vi "Jacobian_h.vi"(1 "State":T1) -> (0 "J_h(H_n)":dbl[](array[numeric]))   [LabVIEW 2019]
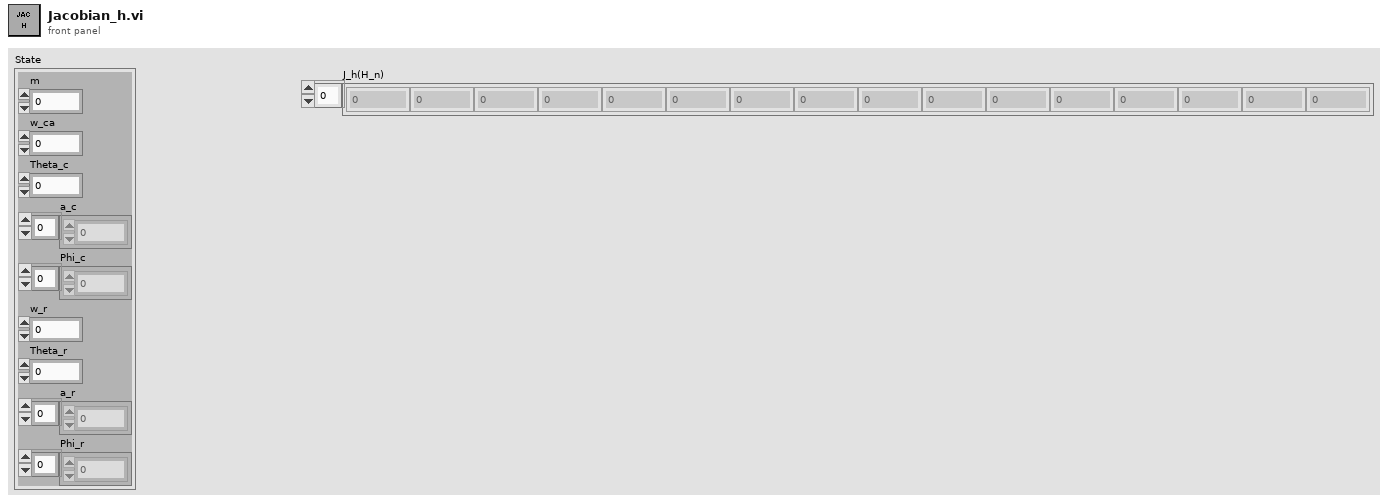
[diagram p1: front panel]
types:
  T1 = cluster{"m":dbl, "w_ca":dbl, "Theta_c":dbl, "a_c":dbl[], "Phi_c":dbl[], "w_r":dbl, "Theta_r":dbl, "a_r":dbl[], "Phi_r":dbl[]}
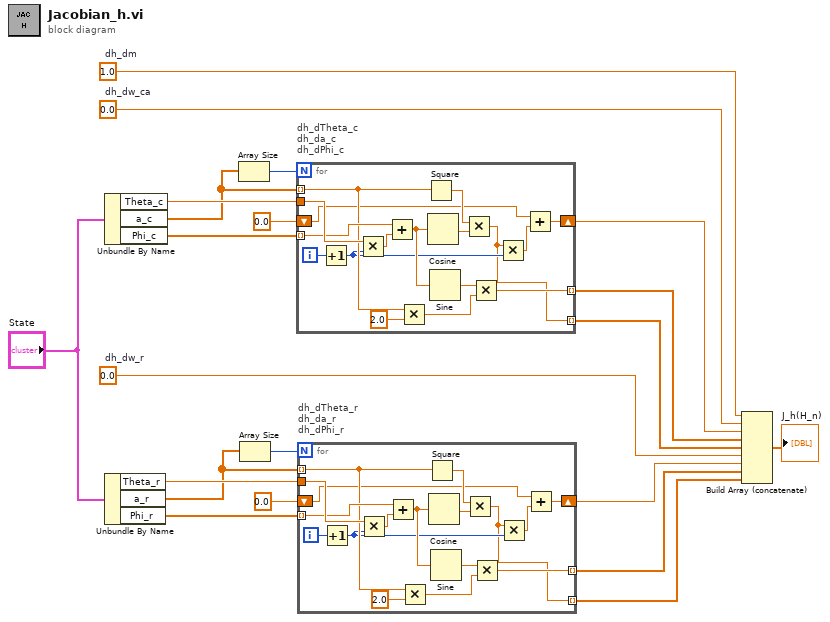
[diagram p0: block diagram]
diagram:
  w11 = 0.0  # dh_dw_r
  w16 = 0.0  # dh_dw_ca
  w17 = 1.0  # dh_dm
  n1 = Unbundle By Name("State") -> ("Theta_c"=w7:dbl, "a_c"=w6:dbl[], "Phi_c"=w5:dbl[])
  n2 = Unbundle By Name("State") -> ("Theta_r"=w3:dbl, "a_r"=w2:dbl[], "Phi_r"=w1:dbl[])
  n3 = Array Size(array=w6) -> (size(s)=w21:i32)
  n4 = Array Size(array=w2) -> (size(s)=w19:i32)
  n5 = for "dh_dTheta_c\ndh_da_c\ndh_dPhi_c" {
    N: w21 -> [_]
    tunnel: w6 -> [w31] mode=indexing
    tunnel: w7 -> [w37]
    tunnel: w5 -> [w36] mode=indexing
    shift-right: [w33] -> w15
    shift-left: 0.0 -> [w27]
    tunnel: [w25] -> w14 mode=indexing
    tunnel: [w22] -> w12 mode=indexing
    i -> [w38]
    n6 = Increment(x=w38) -> (x+1=w24:i32)
    n7 = Multiply(x=w37, y=w24) -> (x*y=w35:dbl)
    n8 = Add(x=w36, y=w35) -> (x+y=w32:dbl)
    n9 = Multiply(x=w31, y=2.0) -> (x*y=w28:dbl)
    n10 = Square(x=w31) -> (x^2=w34:dbl)
    n11 = Cosine(x=w32) -> (cos(x)=w26:dbl)
    n12 = Sine(x=w32) -> (sin(x)=w29:dbl)
    n13 = Multiply(x=w34, y=w26) -> (x*y=w22:dbl)
    n14 = Multiply(x=w29, y=w28) -> (x*y=w25:dbl)
    n15 = Multiply(x=w22, y=w24) -> (x*y=w23:dbl)
    n16 = Add(x=w27, y=w23) -> (x+y=w33:dbl)
  }
  n17 = for "dh_dTheta_r\ndh_da_r\ndh_dPhi_r" {
    N: w19 -> [_]
    tunnel: w2 -> [w48] mode=indexing
    tunnel: w3 -> [w54]
    tunnel: w1 -> [w53] mode=indexing
    shift-right: [w50] -> w10
    shift-left: 0.0 -> [w44]
    tunnel: [w42] -> w9 mode=indexing
    tunnel: [w39] -> w8 mode=indexing
    i -> [w55]
    n18 = Increment(x=w55) -> (x+1=w41:i32)
    n19 = Multiply(x=w54, y=w41) -> (x*y=w52:dbl)
    n20 = Add(x=w53, y=w52) -> (x+y=w49:dbl)
    n21 = Multiply(x=w48, y=2.0) -> (x*y=w45:dbl)
    n22 = Square(x=w48) -> (x^2=w51:dbl)
    n23 = Cosine(x=w49) -> (cos(x)=w43:dbl)
    n24 = Sine(x=w49) -> (sin(x)=w46:dbl)
    n25 = Multiply(x=w51, y=w43) -> (x*y=w39:dbl)
    n26 = Multiply(x=w46, y=w45) -> (x*y=w42:dbl)
    n27 = Multiply(x=w39, y=w41) -> (x*y=w40:dbl)
    n28 = Add(x=w44, y=w40) -> (x+y=w50:dbl)
  }
  n29 = Build Array (concatenate)(w17, w16, w15, w14, w12, w11, w10, w9, w8) -> (→"J_h(H_n)":dbl[])
